vi "Create All Message Queues.vi"(8 "error in":errorcluster) -> (0 "error out":errorcluster, 3 "Message Queues out":T1)   [LabVIEW 2015, in "Message Queue.lvlib"]
doc: "This VI creates and initializes all the message queues for your application. If your application requires more than one message queue, right-click the \"Message Queues\" constant above and select Open Type Def. Add the new Message Queue(s) to the type definition, then initialize them in this VI."
uses:
  Message Queue.lvlib
  All Message Queues.ctl
  Message Cluster.ctl
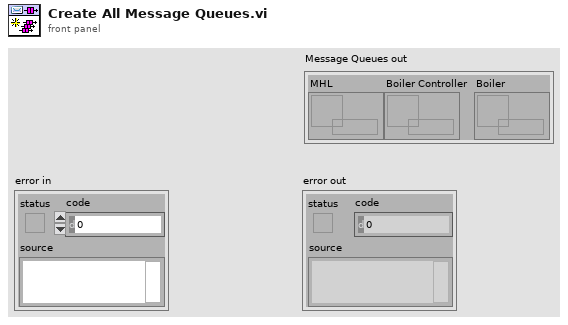
[diagram p1: front panel]
types:
  T1 = typedef "Message Queue.lvlib/All Message Queues.ctl" = cluster{"MHL":refnum<queue>, "Boiler Controller":refnum<queue>, "Boiler ":refnum<queue>}
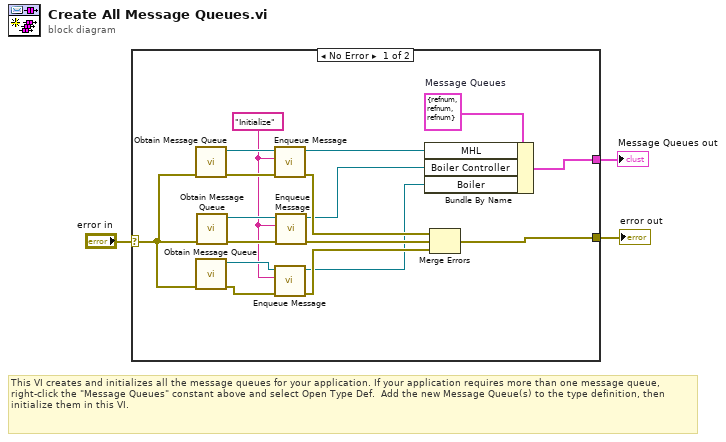
[diagram p0: block diagram]
diagram:
  # "This VI creates and initializes all the message queues for your application. If your application requires more than one message queue, right-click the \"Message Queues\" constant above and select Open Type Def.  Add the new Message Queue(s) to the type definition, then initialize them in this VI."
  n1 = case shown="No Error" "error in" {
    selector: "error in" -> [w9 w21]
    tunnel: [w14 w21] -> w3
    tunnel: [w19 _] -> w2
    frame No Error {
      w5 = "Initialize" ("Message")
      w20 = T1 {"MHL"=refnum, "Boiler Controller"=refnum, "Boiler "=refnum}  # Message Queues
      n2 = call "Obtain Message Queue.vi"("error in (no error)"=w9) -> ("error out"=w18:errorcluster, "Message Queue"=w12:refnum<queue>)  [unwired: 9 in]
      n3 = call "Obtain Message Queue.vi"("error in (no error)"=w9) -> ("error out"=w8:errorcluster, "Message Queue"=w6:refnum<queue>)  [unwired: 9 in]
      n4 = call "Obtain Message Queue.vi"("error in (no error)"=w9) -> ("error out"=w17:errorcluster, "Message Queue"=w10:refnum<queue>)  [unwired: 9 in]
      n5 = call "Enqueue Message.vi"("error in (no error)"=w18, "Message"=w5, "Message Queue"=w12) -> ("error out"=w16:errorcluster, "dup Message Queue"=w11:refnum<queue>)  [unwired: 7 in]
      n6 = call "Enqueue Message.vi"("error in (no error)"=w8, "Message"=w5, "Message Queue"=w6) -> ("error out"=w7:errorcluster, "dup Message Queue"=w4:refnum<queue>)  [unwired: 7 in]
      n7 = call "Enqueue Message.vi"("error in (no error)"=w17, "Message"=w5, "Message Queue"=w10) -> ("error out"=w15:errorcluster, "dup Message Queue"=w13:refnum<queue>)  [unwired: 7 in]
      n8 = Bundle By Name(cluster=w20, "MHL"=w11, "Boiler Controller"=w13, "Boiler"=w4) -> (w19:T1)
      n9 = Merge Errors(w16, w15, w7) -> (w14:errorcluster)
    }
    frame Error {
    }
  }
  "Message Queues out" <- w2
  "error out" <- w3
